vi "GVServos.vi"() -> ()   [LabVIEW 2010]
panel:
  in  "ServosWarmHigh (us)KaltHigh(us)":T1
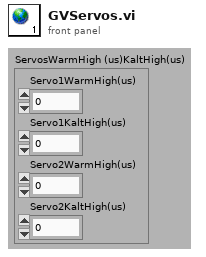
[diagram p1: front panel]
types:
  T1 = cluster{"Servo1WarmHigh(us)":u32, "Servo1KaltHigh(us)":u32, "Servo2WarmHigh(us)":u32, "Servo2KaltHigh(us)":u32}
diagram:
